vi "Filter Data.vi"(6 "Count? (F)":bool, 8 "error in (no error)":errorcluster, 9 "Value Filters[]":cluster{"Header":string, "Value":string}[](array[cluster]), 10 "Header Order[]":string[](array[string]), 11 "SLL Table in":refnum<class "SLL Table.lvclass">) -> (0 "error out":errorcluster, 1 "2D Data Out[][]":string[][](array[string]), 2 "Headers Out[]":string[](array[string]), 3 "SLL Table out":refnum<class "SLL Table.lvclass">)   [LabVIEW 2014, in "SLL Table.lvclass"]
doc: "Get the data that you need & in the column order you want. \n\nYou can specify the column header and the value as conditions."
uses:
  SLL Table.lvclass
  <userlib>/_OpenG.lib/array/array.llb/Remove Duplicates from 1D Array (String)__ogtk.vi
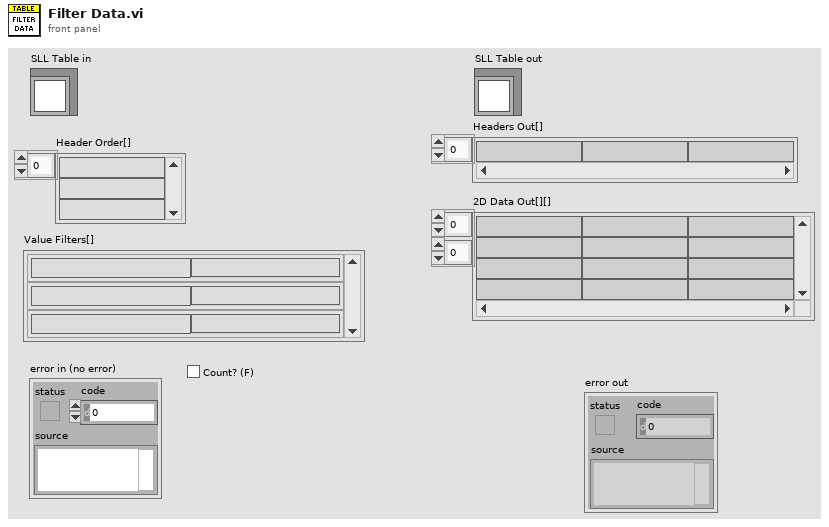
[diagram p1: front panel]
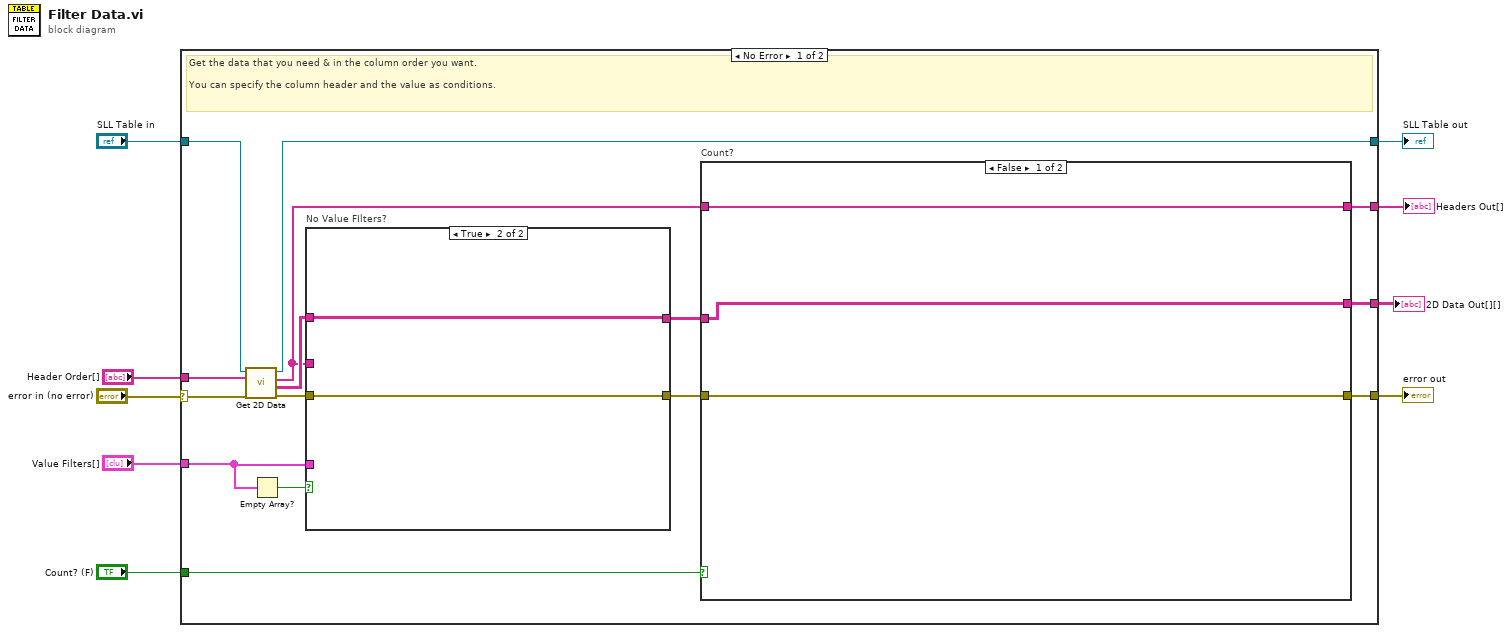
[diagram p0: block diagram]
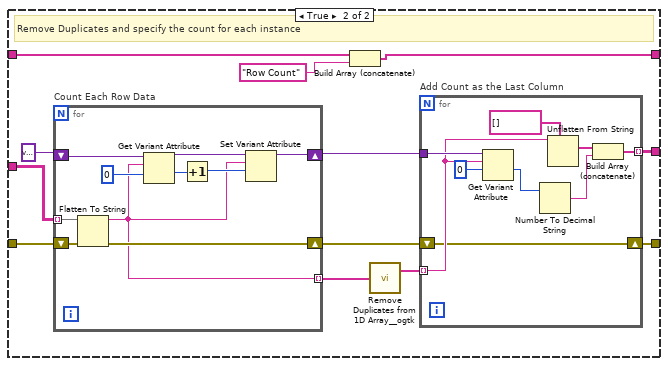
[diagram p2: hidden frame]
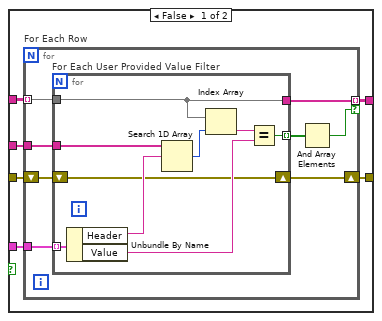
[diagram p3: hidden frame]
diagram:
  n1 = case shown="No Error" "error in (no error)" {
    selector: "error in (no error)" -> [w24 w85]
    tunnel: [w13 w85] -> w8
    tunnel: [w22 w84] -> w6
    tunnel: "SLL Table in" -> [w23 w84]
    tunnel: "Header Order[]" -> [w21 _]
    tunnel: [w20 _] -> w4
    tunnel: [w19 _] -> w3
    tunnel: "Value Filters[]" -> [w16 _]
    tunnel: "Count? (F)" -> [w12 _]
    frame No Error {
      # "Get the data that you need & in the column order you want. \n\nYou can specify the column header and the value as conditions."
      n2 = call "Get 2D Data.vi"("error in (no error)"=w24, "Header Order[]"=w21, "SLL Spreadsheet in"=w23) -> ("error out"=w11:errorcluster, "2D Data Out[][]"=w18:string[][], "Headers Out[]"=w14:string[], "SLL Spreadsheet out"=w22:refnum<class "SLL Table.lvclass">)  [unwired: 5 in]
      n3 = Empty Array?(array=w16) -> (empty?=w17:bool)
      n4 = case "No Value FIlters?" shown="True" w17 {
        tunnel: w18 -> [w64 w83]
        tunnel: w14 -> [w63 _]
        tunnel: w16 -> [w62 _]
        tunnel: [w61 w83] -> w15
        tunnel: w11 -> [w60 w82]
        tunnel: [w59 w82] -> w10
        frame False {
          n5 = for "For Each Row" {
            tunnel: w64 -> [w71] mode=indexing
            tunnel: w63 -> [w70]
            tunnel: w62 -> [w72]
            tunnel: [w69] -> w61 mode=indexing if=w67
            shift-right: [w65] -> w59
            shift-left: w60 -> [w66]
            n6 = for "For Each User Provided Value Filter" {
              tunnel: w72 -> [w81] mode=indexing
              tunnel: w71 -> [w74]
              tunnel: w70 -> [w80]
              tunnel: [w75] -> w68 mode=indexing
              tunnel: [w74] -> w69
              shift-right: [w73] -> w65
              shift-left: w66 -> [w73]
              n7 = Unbundle By Name(w81) -> ("Header"=w79:string, "Value"=w76:string)
              n8 = Search 1D Array(1D array=w80, element=w79) -> (index of element=w78:i32)  [unwired: 1 in]
              n9 = Index Array(array=w74, index=w78) -> (element=w77:string)
              n10 = Equal?(x=w77, y=w76) -> (x = y?=w75:bool)
            }
            n11 = And Array Elements(Boolean array=w68) -> (logical AND=w67:bool)
          }
        }
        frame True {
          # "No Value Filters"
        }
      }
      n12 = case "Count?" shown="False" w12 {
        tunnel: [w27 w36] -> w20
        tunnel: [w26 w35] -> w19
        tunnel: w15 -> [w26 w33]
        tunnel: w14 -> [w27 w32]
        tunnel: [w25 w29] -> w13
        tunnel: w10 -> [w25 w28]
        frame False {
        }
        frame True {
          # "Remove Duplicates and specify the count for each instance"
          n13 = for "Count Each Row Data" {
            shift-right: [w55] -> w38
            shift-left: variant -> [w58]
            tunnel: w33 -> [w54] mode=indexing
            shift-right: [w50] -> w30
            shift-left: w28 -> [w51]
            tunnel: [w49] -> w34 mode=indexing
            n14 = Flatten To String(anything=w54, error in (no error)=w51) -> (data string=w49:string, error out=w50:errorcluster)  [unwired: 2 in, 1 out]
            n15 = Get Variant Attribute(Variant=w58, name=w49, default value (empty Variant)=0) -> (duplicate Variant=w56:variant, value=w53:i32)  [unwired: 1 in, 2 out]
            n16 = Increment(x=w53) -> (x+1=w52:i32)
            n17 = Set Variant Attribute(Variant=w56, name=w49, value=w52) -> (Variant out=w55:variant)  [unwired: 1 in, 2 out]
          }
          n18 = Build Array (concatenate)(w32, "Row Count") -> (w36:string[])
          n19 = call-poly <userlib>:"Remove Duplicates from 1D Array__ogtk.vi"("Input Array"=w34) -> ("Output Array"=w31:string[])  [unwired: 1 out]
          n20 = for "Add Count as the Last Column" {
            tunnel: w38 -> [w48]
            tunnel: w31 -> [w44] mode=indexing
            tunnel: [w41] -> w35 mode=indexing
            shift-right: [w40] -> w29
            shift-left: w30 -> [w40]
            n21 = Get Variant Attribute(Variant=w48, name=w44, default value (empty Variant)=0) -> (value=w46:i32)  [unwired: 1 in, 3 out]
            n22 = Number To Decimal String(number=w46) -> (decimal integer string=w42:string)  [unwired: 1 in]
            n23 = Unflatten From String(type=string[] [] ("2D Data Out[][]"), binary string=w44) -> (value=w43:string[])  [unwired: 3 in, 2 out]
            n24 = Build Array (concatenate)(w43, w42) -> (w41:string[])
          }
        }
      }
    }
    frame Error {
    }
  }
  "error out" <- w8
  "SLL Table out" <- w6
  "2D Data Out[][]" <- w3
  "Headers Out[]" <- w4
